vi "P6.vi"() -> ()   [LabVIEW 2024]
panel:
  out "Hot":bool
  out "Cold":bool
  in  "stop":bool
  out "Vp":dbl
  out "Vdiff":dbl
  out "Temp":dbl
  out "Waveform Chart":dbl(graph)
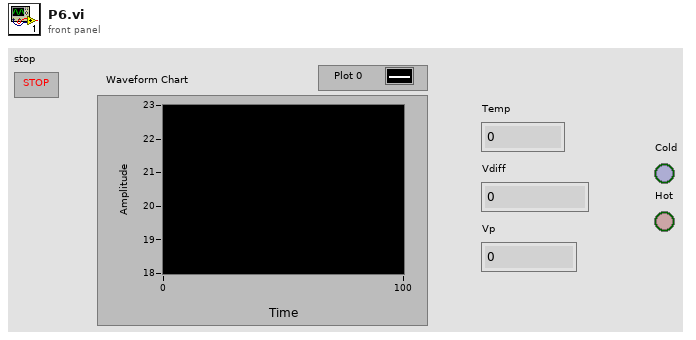
[diagram p1: front panel]
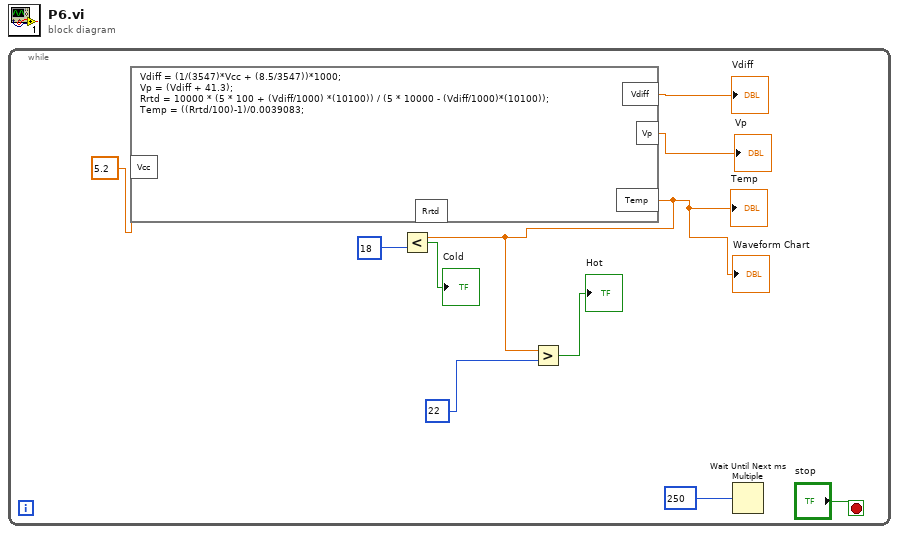
[diagram p0: block diagram]
diagram:
  n1 = while {
    stop <- "stop" stop-if-true
    n2 = formula code="Vdiff = (1/(3547)*Vcc + (8.5/3547))*1000;\nVp = (Vdiff + 41.3);\nRrtd = 10000 * (5 * 100 + (Vdiff/1000) *(10100)) / (5 * 10000 - (Vdiff/1000)*(10100));\nTemp = ((Rrtd/100)-1)/0.0039083;"("Vcc"=5.2) -> ("Vdiff"=→"Vdiff":dbl, "Vp"=→"Vp":dbl, "Temp"=w2:dbl)  [unwired: 1 out]
    "Waveform Chart" <- w2
    "Temp" <- w2
    n3 = Less?(x=w2, y=18) -> (x < y?=→"Cold":bool)
    n4 = Greater?(x=w2, y=22) -> (0:→"Hot":bool)
    n5 = Wait Until Next ms Multiple(millisecond multiple=250) -> ()  [unwired: 1 out]
  }
